vi "ExTestPutRowF32.vi"() -> ()   [LabVIEW 2010]
panel:
  out "Image Display 2":sgl[][](graph)
  out "error out":errorcluster
  in  "error in (no error)":errorcluster
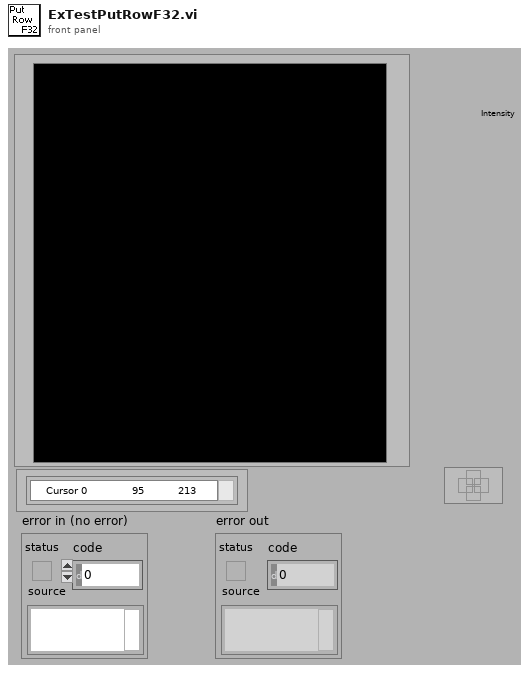
[diagram p1: front panel]
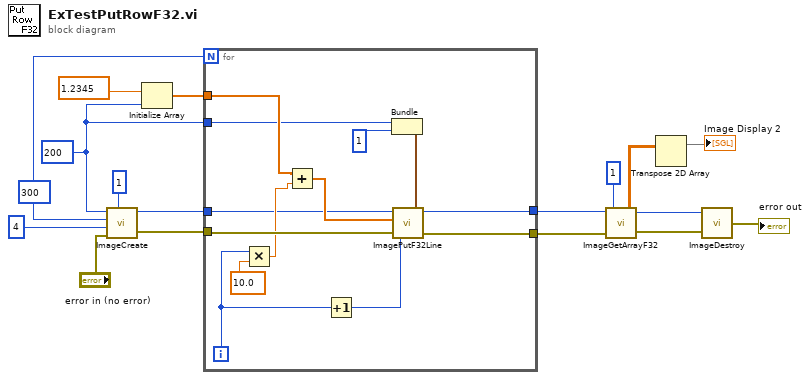
[diagram p0: block diagram]
diagram:
  w4 = 200
  w15 = 300
  n1 = call <userlib>:"ImageCreate.vi"("X dimension"=w4, "Y dimension"=w15, "Data Type"=4, "error in"="error in (no error)", "Number Of Frames"=1) -> ("Image Handle"=w5:u32, "error out"=w7:errorcluster)
  n2 = Initialize Array(1.2345, w4) -> (w6:dbl[])
  n3 = for {
    N: w15 -> [_]
    tunnel: w7 -> [w30]
    tunnel: w6 -> [w25]
    tunnel: w5 -> [w23]
    tunnel: w4 -> [w22]
    tunnel: [w19] -> w3
    tunnel: [w18] -> w1
    i -> [w28]
    n4 = Multiply(x=w28, y=10.0) -> (x*y=w26:dbl)
    n5 = Add(x=w25, y=w26) -> (x+y=w24:dbl[])
    n6 = Increment(x=w28) -> (x+1=w29:i32)
    n7 = Bundle(w22, 1) -> (w20:cluster{i32, i32})  [unwired: 1 in]
    n8 = call <userlib>:"ImagePutF32Line.vi"("Image Handle"=w23, "Image Data"=w24, "Y Position"=w29, "error in (no error)"=w30, "Image dimensions"=w20) -> ("Image Handle"=w18:u32, "error out"=w19:errorcluster)
  }
  n9 = call <userlib>:"ImageGetArrayF32.vi"("error in"=w3, "Z position"=1, "Image Handle"=w1) -> ("error out"=w2:errorcluster, "Array Float 32"=w11:sgl[][], "Image Handle"=w9:u32)
  n10 = Transpose 2D Array(2D array=w11) -> (transposed array=→"Image Display 2":sgl[][])
  n11 = call <userlib>:"ImageDestroy.vi"("error in"=w2, "Data handle"=w9) -> ("error out"=→"error out":errorcluster)
